vi "ScanPolymorphic.vi"   [LabVIEW 2017]
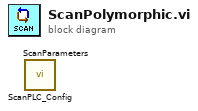
[diagram p0: block diagram]
diagram:
  n1 = call "ScanPLC_Config.vi"() -> ()  [unwired: 11 in, 1 out]
  n2 = call "ScanParameters.vi"() -> ()  [unwired: 11 in, 1 out]
